vi "MinMax x scale.vi"(8 "Error In":errorcluster, 10 "Min Max x Scale]":cluster{dbl, dbl}(slide)={-45.0, 50.0} scale=-80.0..20.0, 11 "Graph In":refnum<vi>) -> (0 "Error Out":errorcluster, 3 "Graph Out":refnum<vi>)   [LabVIEW 2019]
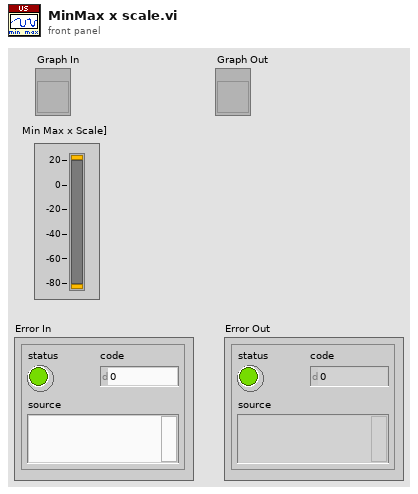
[diagram p1: front panel]
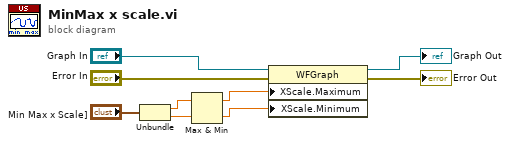
[diagram p0: block diagram]
diagram:
  n1 = Unbundle("Min Max x Scale]") -> (w4:dbl, w5:dbl)
  n2 = Max & Min(x=w4, y=w5) -> (max(x,y)=w2:dbl, min(x,y)=w1:dbl)
  n3 = property on="Property Node" class="WFGraph"(reference="Graph In", error in="Error In", "XScale.Maximum"=w2, "XScale.Minimum"=w1) -> (reference out=→"Graph Out":refnum<vi>, error out=→"Error Out":errorcluster)
